vi "Initialization.vi"(8 "error in":errorcluster) -> (0 "error out":errorcluster)   [LabVIEW 2017]
uses:
  GameConfig/GameConfig_mods.ctl
  Display/Display_mods.ctl
  ManageMovableObjects/ManRef_mods.ctl
  Spaceship/Spaceship_mods.ctl
  Log/Log_mods.ctl
  ManageMovableObjects/HoldData/HoldData_mods.ctl
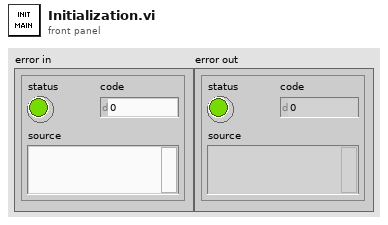
[diagram p1: front panel]
types:
  T1 = typedef "HoldData_mods.ctl" = enum16{"Init", "NewAster", "UpdateAster", "RemoveAster", "GetAsterData", "NewShoot", "UpdateShoot", "RemoveShoot", "GetShootData", "End"}
  T2 = typedef "Log_mods.ctl" = enum16{"Init", "Write", "Clear", "End"}
  T3 = typedef "Spaceship_mods.ctl" = enum16{"Init", "Move", "Rotate", "Translate", "GetData", "End"}
  T4 = typedef "ManRef_mods.ctl" = enum16{"Init", "NewAster", "MoveAll", "DestroyAster", "NewShoot", "DestroyShot", "CheckColision", "End"}
  T5 = typedef "Display_mods.ctl" = enum16{"Init", "GetBase", "DrawAster", "DrawShip", "DrawShoot", "Clear", "Close"}
  T6 = typedef "GameConfig_mods.ctl" = enum16{"Init", "Get"}
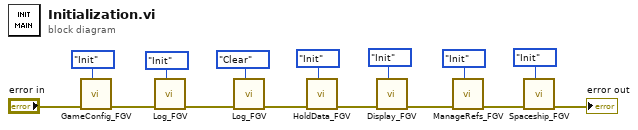
[diagram p0: block diagram]
diagram:
  n1 = call "GameConfig_FGV.vi"("Mods"=GameConfig_mods."Init", "error in"="error in") -> ("error out"=w5:errorcluster)  [unwired: 8 in, 1 out]
  n2 = call "Log_FGV.vi"("Log_mods"=Log_mods."Init", "error in"=w5) -> ("error out"=w6:errorcluster)  [unwired: 9 in]
  n3 = call "Log_FGV.vi"("Log_mods"=Log_mods."Clear", "error in"=w6) -> ("error out"=w3:errorcluster)  [unwired: 9 in]
  n4 = call "HoldData_FGV.vi"("HoldData_mods"=HoldData_mods."Init", "error in"=w3) -> ("error out"=w2:errorcluster)  [unwired: 8 in, 1 out]
  n5 = call "Display_FGV.vi"("Display_mods"=Display_mods."Init", "error in"=w2) -> ("error out"=w12:errorcluster)  [unwired: 8 in, 1 out]
  n6 = call "ManageRefs_FGV.vi"("ManRef_mods"=ManRef_mods."Init", "error in"=w12) -> ("error out"=w11:errorcluster)  [unwired: 9 in]
  n7 = call "Spaceship_FGV.vi"("Spaceship_mods"=Spaceship_mods."Init", "error in"=w11) -> ("error out"=→"error out":errorcluster)  [unwired: 8 in, 1 out]
